vi "Periodic Tasks.vi"(8 "error in":errorcluster) -> ()   [LabVIEW 2014]
doc: "This VI runs in parallel to other tasks. It can contain as many user-defined periodic loops as you need. These can carry out PID or other sorts of timed response."
uses:
  2015-Robot-Code/2015-Robot-Code/2015-Robot-Code/Global Data!!!.vi
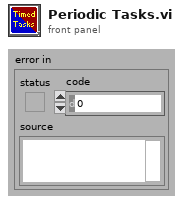
[diagram p1: front panel]
types:
  T1 = typedef "WPI_AccelerometerDevRef.ctl" = cluster{"DevStatus":errorcluster, "Controller":T2, "Scaling":T3, "Analog Channels":T4, "I2C Bus":T6, "SPI Bus":T7, "Accel Range":T8, "ADXL345 Axes":T9, "Handle":i32, "Device Address":u8, "Accel Type":enum16{"Analog", "ADXL345 I2C", "ADXL345 SPI", "Internal"}}
  T2 = typedef "FPGA_TypedefAnalogModule.ctl" = enum16{"Controller 1"}
  T3 = typedef "WPI_AccelerometerScaling.ctl" = cluster{"Gain (VoltsPerG)":dbl, "Center Voltage":dbl}
  T4 = typedef "WPI_AccelerometerAnalogChannels.ctl" = cluster{"X-Axis":T5, "Y-Axis":T5, "Z-Axis":T5}
  T5 = typedef "FPGA_AIChannel.ctl" = enum8{"AI 0", "AI 1", "AI 2", "AI 3", "AI MXP 0", "AI MXP 1", "AI MXP 2", "AI MXP 3", "Invalid"}
  T6 = typedef "i2c_bus.ctl" = enum16{"I2C On-Board", "I2C MXP", "Invalid"}
  T7 = typedef "spi_bus.ctl" = enum16{"SPI On-Board, CS0", "SPI On-Board, CS1", "SPI On-Board, CS2", "SPI On-Board, CS3", "SPI MXP", "Invalid"}
  T8 = typedef "ADXL345 Range.ctl" = u8
  T9 = typedef "WPI_AccelerometerADXL345 Axes.ctl" = cluster{"X-Axis":bool, "Y-Axis":bool, "Z-Axis":bool}
  T10 = cluster{"X-Axis":dbl, "Y-Axis":dbl, "Z-Axis":dbl}
  T11 = typedef "WPI_MotorControlDeviceRef.ctl" = cluster{"DeviceStatus":errorcluster, "Type":T12, "PWM":cluster{"Controller":T13, "PWM Channel":T14, "DeadBand":T15}, "CAN":cluster{"Device Number":u8, "Control Mode":T16, "Semaphore":T17, "Max Vout":dbl, "TalonSRX Control Mode":T18}, "Invert":bool, "TransformRef":T19, "InvTransformRef":T19}
  T12 = typedef "WPI_MotorControlType.ctl" = enum16{"PWM", "CAN", "CANTalonSRX"}
  T13 = typedef "FPGA_TypedefDigitalModule.ctl" = enum16{"Controller 1"}
  T14 = typedef "FPGA_DIOPWMChannel.ctl" = enum8{"PWM 0", "PWM 1", "PWM 2", "PWM 3", "PWM 4", "PWM 5", "PWM 6", "PWM 7", "PWM 8", "PWM 9", "PWM MXP 0", "PWM MXP 1", "PWM MXP 2", "PWM MXP 3", "PWM MXP 4", "PWM MXP 5", "PWM MXP 6", "PWM MXP 7", "PWM MXP 8", "PWM MXP 9", "Invalid"}
  T15 = typedef "WPI_PWMDeadband.ctl" = cluster{"Name":string, "maxPositivePwm":i32, "minPositivePwm":i32, "centerPwm":i32, "maxNegativePwm":i32, "minNegativePwm":i32, "angularRange":u16}
  T16 = typedef "WPI_CANJaguar_ControlMode.ctl" = enum8{"Percent VBus", "Current", "Speed", "Position", "Voltage"}
  T17 = typedef "Semaphore RefNum" = refnum<k1>
  T18 = typedef "WPI_CANTalonSRX_APIControlMode.ctl" = enum8{"Percent VBus", "Speed", "Position", "Slave", "Unchanged / Invalid"}
  T19 = typedef "WPI_PWMTransform_ConPane.ctl" = refnum<vi>
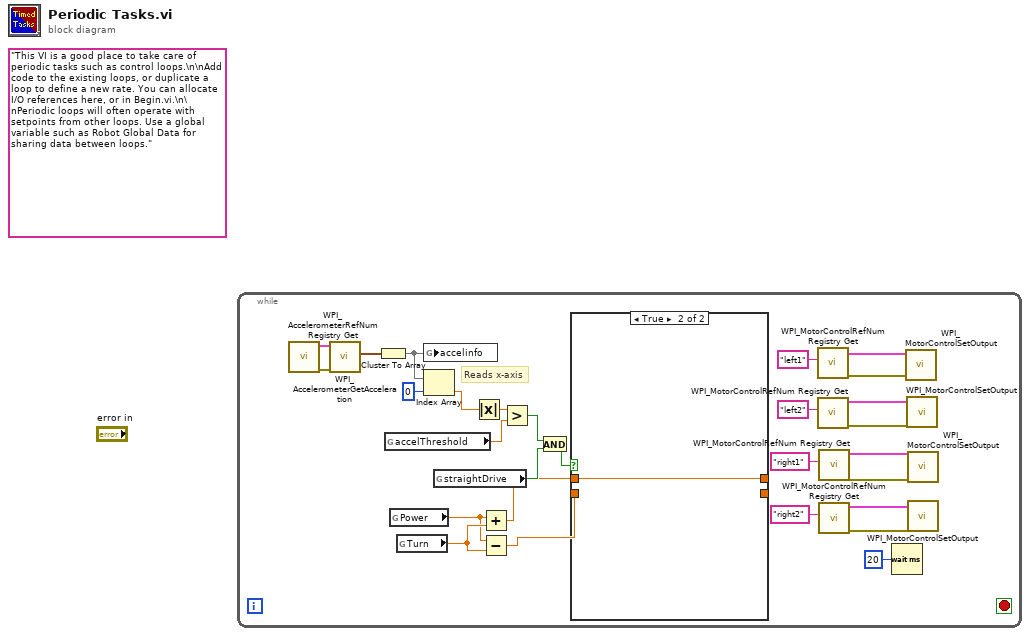
[diagram p0: block diagram]
diagram:
  (unwired) "This VI is a good place to take care of periodic tasks such as control loops.\n\nAdd code to the existing loops, or duplicate a loop to define a new rate. You can allocate I/O references here, or in Begin.vi.\n\nPeriodic loops will often operate with setpoints from other loops. Use a global variable such as Robot Global Data for sharing data between loops."
  n1 = while {
    stop <- _ stop-if-true
    # "Reads x-axis"
    n2 = call <vilib>:"WPI_AccelerometerRefNum Registry Get.vi"() -> ("error out"=w28:errorcluster, "AccelerometerDevRef"=w27:T1)  [unwired: 10 in]
    n3 = call <vilib>:"WPI_AccelerometerGetAcceleration.vi"("error in"=w28, "AccelerometerDevRef"=w27) -> ("Accelerations"=w26:T10)  [unwired: 7 in, 2 out]
    n4 = Cluster To Array(cluster=w26) -> (array=w25:dbl[])
    n5 = global read "Global Data!!!.vi" "accelThreshold"() -> (w21:dbl)
    n6 = global read "Global Data!!!.vi" "Power"() -> (w16:dbl)
    n7 = global read "Global Data!!!.vi" "Turn"() -> (w17:dbl)
    n8 = global write "Global Data!!!.vi" "accelinfo"(w25) -> ()
    n9 = Index Array(array=w25, index=0) -> (element=w22:dbl)
    n10 = global read "Global Data!!!.vi" "straightDrive"() -> (w19:bool)
    n11 = Absolute Value(x=w22) -> (abs(x)=w23:dbl)
    n12 = Add(x=w16, y=w17) -> (x+y=w15:dbl)
    n13 = Subtract(x=w16, y=w17) -> (x-y=w14:dbl)
    n14 = Greater?(x=w23, y=w21) -> (0:w20:bool)
    n15 = And(x=w20, y=w19) -> (x .and. y?=w18:bool)
    n16 = case shown="True" w18 {
      tunnel: w15 -> [w30 w31]
      tunnel: w14 -> [w29 _]
      tunnel: [w30 w31] -> _
      tunnel: [w29 _] -> _
      frame False {
      }
      frame True {
      }
    }
    n17 = call <vilib>:"WPI_MotorControlRefNum Registry Get.vi"("refnum name"="left1") -> ("error out"=w11:errorcluster, "MotorControlDevRef"=w6:T11)  [unwired: 9 in]
    n18 = call <vilib>:"WPI_MotorControlRefNum Registry Get.vi"("refnum name"="left2") -> ("error out"=w12:errorcluster, "MotorControlDevRef"=w7:T11)  [unwired: 9 in]
    n19 = call <vilib>:"WPI_MotorControlRefNum Registry Get.vi"("refnum name"="right1") -> ("error out"=w10:errorcluster, "MotorControlDevRef"=w8:T11)  [unwired: 9 in]
    n20 = call <vilib>:"WPI_MotorControlRefNum Registry Get.vi"("refnum name"="right2") -> ("error out"=w13:errorcluster, "MotorControlDevRef"=w9:T11)  [unwired: 9 in]
    n21 = Wait (ms)(milliseconds to wait=u32 20) -> ()  [unwired: 1 out]
    n22 = call <vilib>:"WPI_MotorControlSetOutput.vi"("error in (no error)"=w11, "MotorControlDevRef"=w6) -> ()  [unwired: 7 in, 3 out]
    n23 = call <vilib>:"WPI_MotorControlSetOutput.vi"("error in (no error)"=w12, "MotorControlDevRef"=w7) -> ()  [unwired: 7 in, 3 out]
    n24 = call <vilib>:"WPI_MotorControlSetOutput.vi"("error in (no error)"=w10, "MotorControlDevRef"=w8) -> ()  [unwired: 7 in, 3 out]
    n25 = call <vilib>:"WPI_MotorControlSetOutput.vi"("error in (no error)"=w13, "MotorControlDevRef"=w9) -> ()  [unwired: 7 in, 3 out]
  }
